vi "GetControlLoopCount.vi"(0 "Handle":u32) -> (7 "FT_Status":u32(ring) items=["FT_OK", "FT_INVALID_HANDLE", "FT_DEVICE_NOT_FOUND", "FT_DEVICE_NOT_OPENED", "FT_IO_ERROR", "FT_INSUFFICIENT_RESOURCES", "FT_INVALID_PARAMETER", "FT_INVALID_BAUD_RATE", "FT_DEVICE_NOT_OPENED_FOR_ERASE", "FT_DEVICE_NOT_OPENED_FOR_WRITE", "FT_FAILED_TO_WRITE_DEVICE", "FT_EEPROM_READ_FAILED", "FT_EEPROM_WRITE_FAILED", "FT_EEPROM_ERASE_FAILED", "FT_EEPROM_NOT_PRESENT", "FT_EEPROM_NOT_PROGRAMMED", "FT_INVALID_ARGS", "FT_NOT_SUPPORTED", "FT_OTHER_ERROR"], 9 "Control Loop Count":i32)   [LabVIEW 2013]
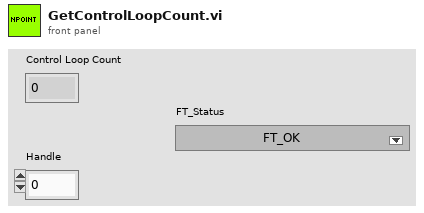
[diagram p1: front panel]
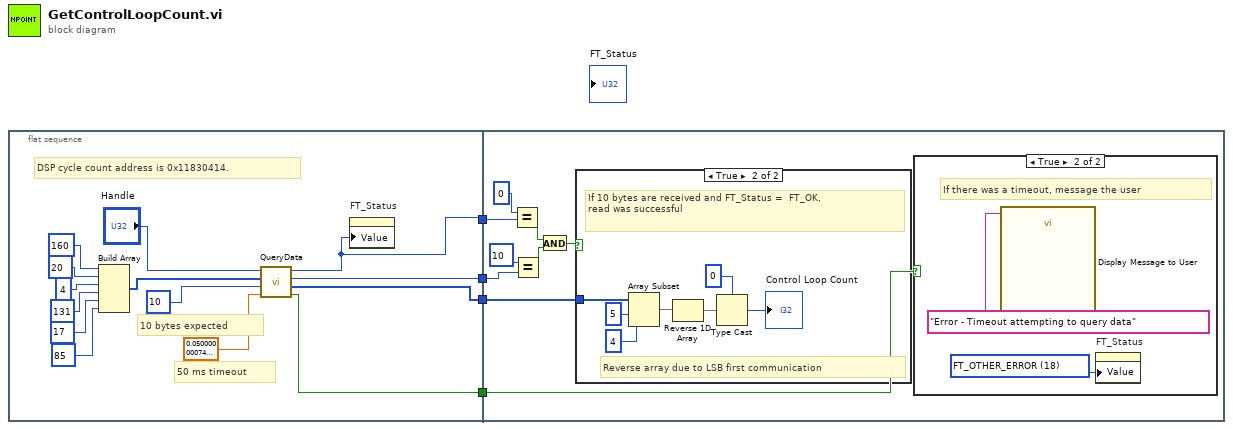
[diagram p0: block diagram]
diagram:
  n1 = flat-sequence {
    tunnel: [w9] -> w4
    tunnel: [w8] -> w3
    tunnel: [w7] -> w2
    tunnel: [w6] -> w1
    tunnel: w4 -> [w27]
    tunnel: w3 -> [w25]
    tunnel: w2 -> [w24]
    tunnel: w1 -> [w22]
    frame #0 {
      # "10 bytes expected"
      # "50 ms timeout"
      # "DSP cycle count address is 0x11830414."
      n2 = Build Array(u8 160 ("element"), u8 20 ("element"), u8 4 ("element"), u8 131 ("element"), u8 17 ("element"), u8 85 ("element")) -> (w12:u8[])
      n3 = call "QueryData.vi"("TimeoutLengthSeconds"=sgl 0.05, "NumBytesExpected"=u32 10, "Message"=w12, "Handle"="Handle") -> ("Timeout"=w7:bool, "Return Array"=w8:u8[], "Bytes Read"=w9:u32, "FT_Status"=w6:u32)  [unwired: 4 in]
      n4 = property on="FT_Status" class="Ring (strict)"("Value"=w6) -> ()  [unwired: 2 in, 2 out]
    }
    frame #1 {
      n5 = Equal?(x=u32 0, y=w22) -> (x = y?=w20:bool)
      n6 = Equal?(x=u32 10, y=w27) -> (x = y?=w21:bool)
      n7 = And(x=w20, y=w21) -> (x .and. y?=w19:bool)
      n8 = case shown="True" w19 {
        tunnel: w25 -> [_ w36]
        frame False {
        }
        frame True {
          # "Reverse array due to LSB first communication"
          # "If 10 bytes are received and FT_Status =  FT_OK,\nread was successful"
          n9 = Array Subset(array=w36, index=5, length=4) -> (w32:u8[])
          n10 = Reverse 1D Array(array=w32) -> (reversed array=w31:u8[])
          n11 = Type Cast(type=0, x=w31) -> (*(type *) &x=→"Control Loop Count":i32)
        }
      }
      n12 = case shown="True" w24 {
        frame False {
        }
        frame True {
          w28 = u32 18 items=["FT_OK", "FT_INVALID_HANDLE", "FT_DEVICE_NOT_FOUND", "FT_DEVICE_NOT_OPENED", "FT_IO_ERROR", "FT_INSUFFICIENT_RESOURCES", "FT_INVALID_PARAMETER", "FT_INVALID_BAUD_RATE", "FT_DEVICE_NOT_OPENED_FOR_ERASE", "FT_DEVICE_NOT_OPENED_FOR_WRITE", "FT_FAILED_TO_WRITE_DEVICE", "FT_EEPROM_READ_FAILED", "FT_EEPROM_WRITE_FAILED", "FT_EEPROM_ERASE_FAILED", "FT_EEPROM_NOT_PRESENT", "FT_EEPROM_NOT_PROGRAMMED", "FT_INVALID_ARGS", "FT_NOT_SUPPORTED", "FT_OTHER_ERROR"] ("FT_Status")
          # "If there was a timeout, message the user"
          n13 = call "Display Message to User"("Message"="Error - Timeout attempting to query data") -> ()  [unwired: 9 in, 2 out]
          n14 = property on="FT_Status" class="Ring (strict)"("Value"=w28) -> ()  [unwired: 2 in, 2 out]
        }
      }
    }
  }
